vi "Pack Message.vi"(8 "error in (no error)":errorcluster, 11 "Message Boolean in":refnum<class "Message Boolean.lvclass">) -> (0 "error out":errorcluster, 1 "Packed Message":string, 2 "Message Name":string, 3 "Message Boolean out":refnum<class "Message Boolean.lvclass">)   [LabVIEW 2016, in "Stream Mediator.lvlib" / "Message Boolean.lvclass"]
uses:
  <userlib>/Composed Systems/Stream/Mediator/Classes/Message Boolean/Message Boolean.lvclass
  C:/Program Files (x86)/National Instruments/LabVIEW 2016/user.lib/Composed Systems/Stream/Mediator/Classes/Message Interface/Message Interface.lvclass
  <userlib>/Composed Systems/Stream/Mediator/Classes/Message Boolean/Message Boolean.lvclass/Message Boolean.ctl
  <userlib>/Composed Systems/Stream/Mediator/Classes/Message Interface/Message Interface.lvclass
  <vilib>/addons/_JKI.lib/Serialization/JSON/JKI JSON Serialization.lvlib
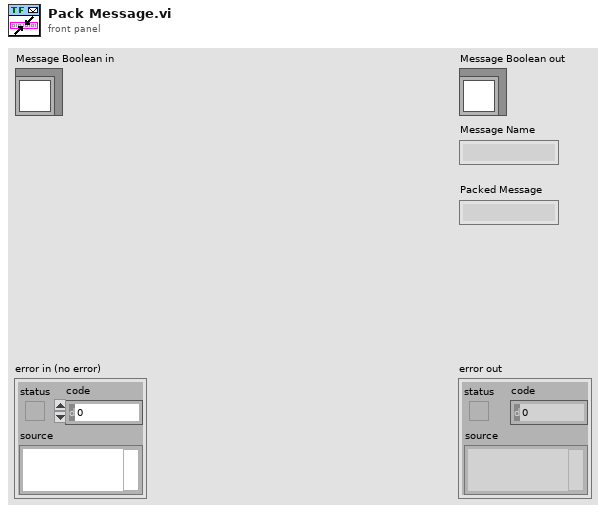
[diagram p1: front panel]
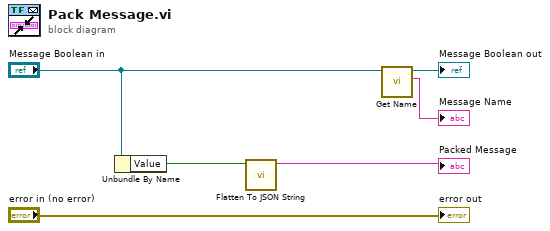
[diagram p0: block diagram]
diagram:
  n1 = Unbundle By Name("Message Boolean in") -> ("Value"=w3:bool)
  n2 = call <vilib>:"Flatten To JSON String.vi"("Variant"=w3) -> ("JSON String"=→"Packed Message":string)  [unwired: 9 in, 1 out]
  n3 = call <userlib>:"Get Name.vi"("Message Interface in"="Message Boolean in") -> ("Name"=→"Message Name":string, "Message Interface out"=→"Message Boolean out":refnum<class "Message Boolean.lvclass">)  [unwired: 8 in, 1 out]
  "error out" <- "error in (no error)"
